vi "4_2_PTLF_Classification_Inference(FPGA).vi"() -> ()   [LabVIEW 2020]
uses:
  <vilib>/userDefined/High Color/nirio_resource_hc.ctl
  <vilib>/FPGAPlugInAG/Dynamic/niLvFpga_Download_Dynamic.vi
  <vilib>/FPGAPlugInAG/Dynamic/niLvFpga_Run_Dynamic.vi
  <vilib>/Ngene/DeepLTK FPGA Addon/Toolkit/NNF_Host/API/NNF_Set_Input/NNF_Set_Input(1D_I8).vi
  <vilib>/rvi/interface/nirviMethod/nirviMethod.xnode
  <vilib>/Ngene/Deep Learning Toolkit/Toolkit/Deep_Learning_Toolkit_by_Ngene.lvlib
  <vilib>/measure/NI_MABase.lvlib
  <vilib>/Ngene/DeepLTK FPGA Addon/Toolkit/DeepLTK_FPGA_Addon.lvlib
  <vilib>/ptbypt/NI_PtbyPt.lvlib
panel:
  in  "Force CPU(All)?":bool
  out "error out 2":errorcluster
  out "Inference Time":dbl=0.08973853333413394 format="%#_3p"
  in  "FPGA Bitfile":path=path "D:/Ngene/GitHub/deepltk_fpga_examples/FPGA Bitfiles/NNF_sbRIO_9609_8Cores_120MHz.lvbitx"
  in  "FPGA target":T1="rio://10.0.0.39/RIO0" caption="RIO Device"
  out "Loop Time":dbl=1506.7505208222221 format="%#_3p"
  in  "Scalers File Path":path=path "D:/Ngene/GitHub/deepltk_fpga_examples/3_PTLF_Classification(PXI,sbRIO)/Models/1_PTLF_Classification_Converted/NNF_ptlf_classifier_net_scalers_24_11_21__13_54_07.cfg"
  in  "Position":dbl(slide)=0.4116719242902208 scale=0.0..1.0
  in  "Fault Generation":T2(tab)=enum."Transient"
  in  "scale":sgl(slide)=0.65833336 scale=0.5..0.7
  in  "Duration(#s)":i32(slide)=388 scale=200.0..600.0
  in  "scale":sgl(slide)=1.4484375 scale=1.35..1.5
  in  "Duration(#s)":i32(slide)=403 scale=200.0..600.0
  in  "Duration(#s)":i32(slide)=366 scale=200.0..600.0
  in  "Tau":dbl(slide)=337.5 scale=200.0..600.0
  in  "Frequency":dbl(slide)=1666.6666666666665 scale=1000.0..2000.0
  in  "Amplitude":dbl(slide)=184.375 scale=150.0..200.0
  in  "Offset":sgl(slide)=105.208336 scale=50.0..150.0
  in  "Duration(#s)":i32(slide)=449 scale=200.0..600.0
  out "Predicted Class":string="Transient"
  out "Class Labels":string[](array[string])=["DC Offset", "Interruption", "Normal", "Sag", "Swell", "Transient"]
  out "Generated WaveForm":waveform(sgl)(graph)={"t0"=timestamp(0 s since 1904-01-01), "dt"=1.0, "Y"=array[2000 elements]}
  in  "Weight File Path":path=path "D:/Ngene/GitHub/deepltk_fpga_examples/3_PTLF_Classification(PXI,sbRIO)/Models/1_PTLF_Classification_Converted/NNF_ptlf_classifier_weights_24_11_21__13_54_07.bin"
  in  "Configuration File Path":path=path "D:/Ngene/GitHub/deepltk_fpga_examples/3_PTLF_Classification(PXI,sbRIO)/Models/1_PTLF_Classification_Converted/NNF_ptlf_classifier_net_cfg_24_11_21__13_54_07.cfg"
  out "Class Probabilities":sgl[](array[slide])=[3.9739523e-05, 7.152872e-06, 1.9828617e-07, 5.2368828e-06, 1.1418055e-05, 0.9999362] scale=0.0..1.0
  in  "Stop":bool
  # "Overview: Demonstrates the usage of DeepLTK FPGA Addon for loading the model pretrained for Power Line Fault Classification and running for inference on FPGA.\nRequirements: \n• DeepLTK - Deep Learning Toolkit for LabVIEW (https://www.ngene.co/deep-learning-toolkit-for-labview)\n• DeepLTK FPGA Addon (https://www.ngene.co/deepltk-accelerator-for-fpga)\nInstructions:\nNote: To run the example on an RT target, copy the converted model to the RT target.\n1. Select FPGA target at FPGA Target control. PXI or remote sbRIO FPGA target can be specified.\n2. Provide path to compiled FPGA bitfile at FPGA Bitfile control. A sample is available in the \"Examples\\FPGA Bitfiles\" folder.\n3. Provide paths to .cfg, .bin and scalers.cfg files generated during model conversion or sample from project (located in \"Models\\1_PTLF_Classification_Converted\" folder)\nat Network Configuration File Path, Weight File Path and Scalers File Path controls.\n4. Run the VI\n5. Choose type of the fault and change the parameters and observe the predicted type of the fault.\n6. Press the Stop button to stop the VI.\nMore Examples: https://github.com/ngenehub/deepltk_fpga_examples"
  # "Power Transmission Line Fault Classification - Inference on FPGA"
  # "Copy resource path from NI MAX if needed"
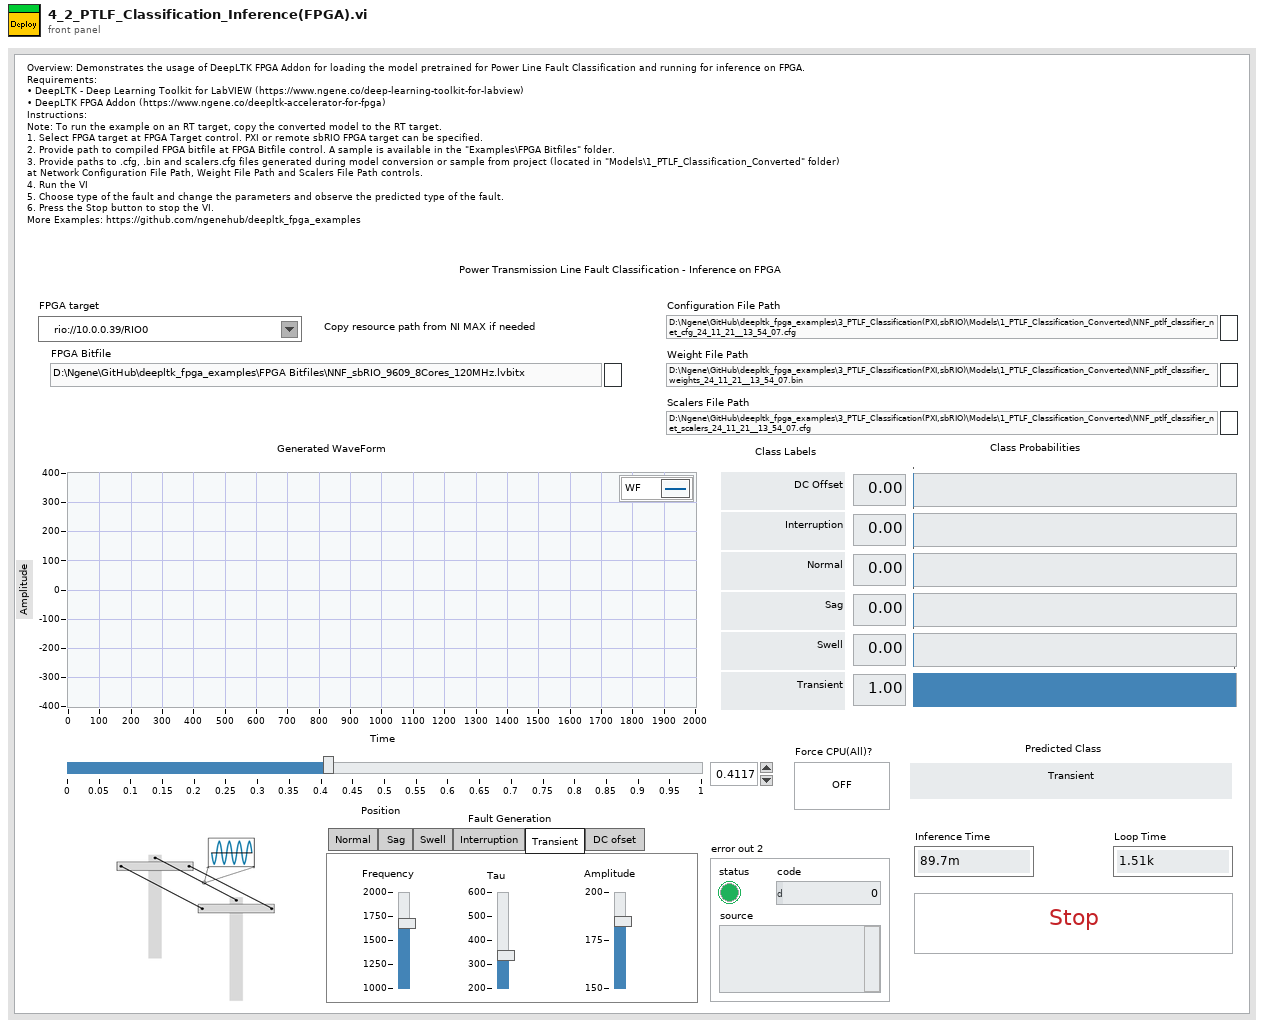
[diagram p1: front panel]
types:
  T1 = typedef "nirio_resource_hc.ctl" = tag
  T2 = enum32{"Normal", "Sag ", "Swell", "Interruption", "Transient", "DC ofset "}
  T3 = typedef "DeepLTK_FPGA_Addon.lvlib/NNF.ctl" = cluster{"FPGA VI Ref ":refnum<k20>, "Subnets":T4[], "Dims_In":T6, "#Cores(enum)":T7, "NN_Ref":T8}
  T4 = typedef "DeepLTK_FPGA_Addon.lvlib/NNF_Subnet.ctl" = cluster{"Subnet Type":T5, "Subnet Data":variant, "Input Scaler":sgl, "Output Scaler":sgl}
  T5 = typedef "DeepLTK_FPGA_Addon.lvlib/NNF_Subnet_Type.ctl" = enum16{"CPU", "FPGA", "Split FPGA"}
  T6 = typedef "Deep_Learning_Toolkit_by_Ngene.lvlib/NN_Dims(C,H,W).ctl" = cluster{"C":i32, "H":i32, "W":i32}
  T7 = typedef "DeepLTK_FPGA_Addon.lvlib/NNF_No_Of_Cores.ctl" = enum16{"4CH", "8CH"}
  T8 = typedef "DeepLTK_FPGA_Addon.lvlib/NN_DVR.ctl" = refnum<data-value>
  T9 = typedef "Deep_Learning_Toolkit_by_Ngene.lvlib/NN_Layer.ctl" = cluster{"Name":string, "Layer_Data":variant, "Layer_Type":T10, "Dims_In":T6, "Layers_In":variant, "Dims_Out":T6, "Layers_Out":variant, "Metrics":T11, "GPU_Data":variant, "mBatch":i32, "NN_Device":T12, "NNg_hdls":T13, "Train?":bool, "Dimty":T14, "RecptField":T15}
  T10 = typedef "Deep_Learning_Toolkit_by_Ngene.lvlib/NN_Layer_Type.ctl" = enum16{"Input1D", "Input3D", "Conv1D", "Conv2D", "Conv2D_Adv", "MaxPool", "AvgPool", "UpSample", "DropOut3D", "ShortCut", "Concat", "SoftMax3D", "FC", "DropOut", "Softmax", "Flatten", "YOLO_v2", "YOLO_v4", "Activation", "BatchNormalization", "Unsupported"}
  T11 = typedef "Deep_Learning_Toolkit_by_Ngene.lvlib/NN_Layer_Metrics.ctl" = cluster{"Data":dbl, "Params":dbl, "Ops":dbl}
  T12 = typedef "Deep_Learning_Toolkit_by_Ngene.lvlib/NN_Device.ctl" = enum16{"CPU", "GPU"}
  T13 = typedef "Deep_Learning_Toolkit_by_Ngene.lvlib/nng_cuda_handles.ctl" = cluster{"cudnn":u64, "cublas":u64, "stream":u64, "curand":u64}
  T14 = typedef "Deep_Learning_Toolkit_by_Ngene.lvlib/NN_Layer_Dimty.ctl" = enum16{"1D", "3D"}
  T15 = typedef "Deep_Learning_Toolkit_by_Ngene.lvlib/NN_Layer_RF_State.ctl" = cluster{"Dims":T16, "J":T16}
  T16 = typedef "Deep_Learning_Toolkit_by_Ngene.lvlib/NN_Dims(V,H).ctl" = cluster{"V":i32, "H":i32}
  T17 = typedef "Deep_Learning_Toolkit_by_Ngene.lvlib/NN.ctl" = cluster{"Name":string, "No of Layers":i32, "mBatch":i32, "Layers":T18[], "Dimty":T19, "Dims_In":T6, "Dims_Out":T6, "Working_Dir":path, "Train?":bool, "Train_Params":T20, "LR_Update_Policy":T23, "Session Data":T25, "Ground_truth":T26, "NNg_hdls":T13, "NN_Device":T12, "GPU Id":i32, "Labels":string[], "Receptive Field":T16[], "Loss_Type":T27, "Loss_Cfg_Prms":variant, "NNG_WS":T28}
  T18 = typedef "Deep_Learning_Toolkit_by_Ngene.lvlib/NN_Layer_ref.ctl" = refnum<data-value>
  T19 = typedef "Deep_Learning_Toolkit_by_Ngene.lvlib/NN_In_Out_Dim-ty.ctl" = enum8{"In1D_Out1D", "In3D_Out1D", "In3D_Out3D", "In3D_OutBBox"}
  T20 = typedef "Deep_Learning_Toolkit_by_Ngene.lvlib/NN_Train_Params.ctl" = cluster{"Optimizer":T21, "Beta_1":sgl, "Beta_2":sgl, "Weight Decay(L1)":sgl, "Weight Decay(L2)":sgl, "Data_Sampling":T22}
  T21 = typedef "Deep_Learning_Toolkit_by_Ngene.lvlib/NN_Train_Optimizer.ctl" = enum16{"SGD", "Adam", "Adagrad", "Adadelta", "RMSProp", "Nesterov"}
  T22 = typedef "Deep_Learning_Toolkit_by_Ngene.lvlib/NN_Train_Data_Sampling.ctl" = enum16{"Random", "Sequential"}
  T23 = typedef "Deep_Learning_Toolkit_by_Ngene.lvlib/NN_LR_Policy_Cfg.ctl" = cluster{"Policy_Type":T24, "LR0":dbl, "k":sgl, "WarmUp_Policy":enum16{"Step", "Ramp"}, "WarmUp_Iter":i32, "WarmUp_Ratio":sgl}
  T24 = typedef "Deep_Learning_Toolkit_by_Ngene.lvlib/NN_LR_Policy_Type.ctl" = enum16{"Manual", "Step", "Exp", "1/t"}
  T25 = typedef "Deep_Learning_Toolkit_by_Ngene.lvlib/NN_Train_Session_Data.ctl" = cluster{"Epochs":sgl, "Tot_Iter":i32, "LR":sgl, "LR_iter":i32}
  T26 = typedef "Deep_Learning_Toolkit_by_Ngene.lvlib/NN_Ground_truth.ctl" = cluster{"Y":variant}
  T27 = typedef "Deep_Learning_Toolkit_by_Ngene.lvlib/NN_Loss_Type.ctl" = enum16{"None", "MSE", "CrossEntropy", "YOLO_v2", "YOLO_v4"}
  T28 = typedef "Deep_Learning_Toolkit_by_Ngene.lvlib/NNG_WS.ctl" = cluster{"NNG_WS_Mem":T29, "Max_WS_Size":i64}
  T29 = typedef "Deep_Learning_Toolkit_by_Ngene.lvlib/NNg_WS_Mem_DVR.ctl" = refnum<data-value>
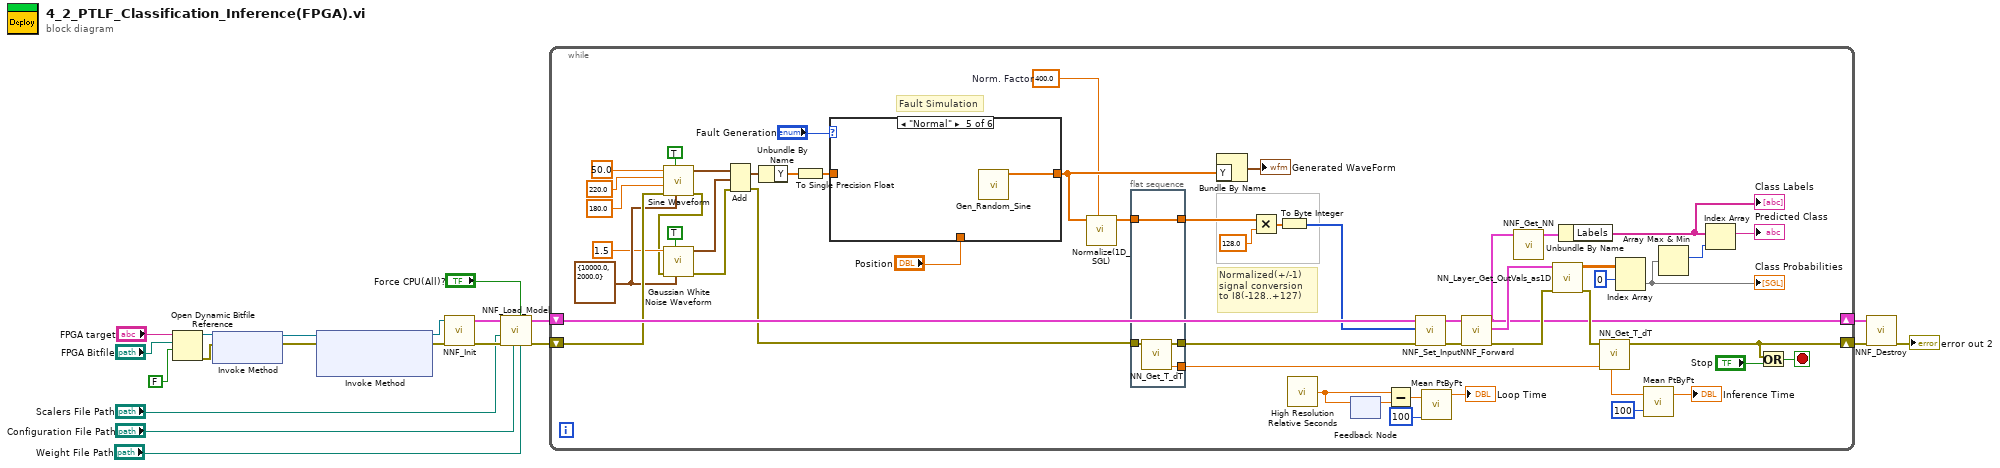
[diagram p0: block diagram]
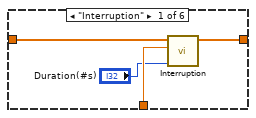
[diagram p2: hidden frame]
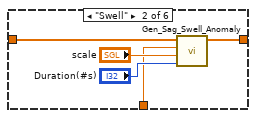
[diagram p3: hidden frame]
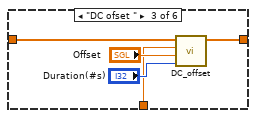
[diagram p4: hidden frame]
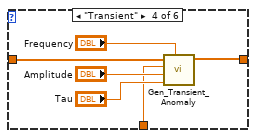
[diagram p5: hidden frame]
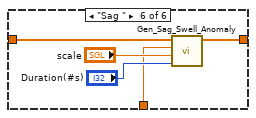
[diagram p6: hidden frame]
diagram:
  n1 = Open Dynamic Bitfile Reference(0:"FPGA target", 1:"FPGA Bitfile", 2:FALSE ("Run When Loaded")) -> (5:w14:refnum<k20>, 8:w9:errorcluster)  [unwired: 2 in]
  n2 = xnode "Invoke Method"("FPGA VI Reference In"=w14, "error in"=w9) -> ("FPGA VI Reference Out"=w13:refnum<k20>, "error out"=w12:errorcluster)
  n3 = xnode "Invoke Method"("FPGA VI Reference In"=w13, "error in"=w12) -> ("FPGA VI Reference Out"=w11:refnum<k20>, "error out"=w10:errorcluster)  [unwired: 1 in]
  n4 = call <vilib>:"NNF_Init.vi"("error in"=w10, "FPGA Interface"=w11) -> ("error out"=w18:errorcluster, "NNF out"=w17:T3)  [unwired: 7 in, 1 out]
  n5 = call <vilib>:"NNF_Load_Model.vi"("Weight File Path"="Weight File Path", "Force CPU(All)?"="Force CPU(All)?", "Network CFG File Path"="Configuration File Path", "Error in"=w18, "Scalers"="Scalers File Path", "NNF in"=w17) -> ("error Out"=w7:errorcluster, "NNF out"=w8:T3)  [unwired: 4 in]
  n6 = while {
    shift-right: [w30] -> w20
    shift-left: w7 -> [w54]
    shift-right: [w23] -> w19
    shift-left: w8 -> [w67]
    stop <- w31 stop-if-true
    w38 = sgl 400.0  # Norm. Factor
    w52 = cluster{"Fs":dbl, "#s":dbl} {"Fs"=10000.0, "#s"=2000.0} ("sampling info")
    # "Normalized(+/-1) signal conversion\nto I8(-128..+127)"
    # "Fault Simulation"
    n7 = call <vilib>:"Sine Waveform.vi"("sampling info"=w52, "reset signal"=TRUE, "error in (no error)"=w54, "phase"=180.0, "amplitude"=220.0, "frequency"=50.0) -> ("error out"=w48:errorcluster, "signal out"=w62:waveform(dbl))  [unwired: 4 in]
    n8 = call <vilib>:"Gaussian White Noise Waveform.vi"("sampling info"=w52, "reset signal"=TRUE, "error in (no error)"=w48, "standard deviation"=sgl 1.5 ("Noise Standart Deviation")) -> ("error out"=w47:errorcluster, "signal out"=w37:waveform(dbl))  [unwired: 6 in]
    n9 = Add(1:w37, 2:w62, 4:w47) -> (0:w50:waveform(dbl), 3:w33:errorcluster)
    n10 = Unbundle By Name(w50) -> ("Y"=w61:dbl[])
    n11 = To Single Precision Float(number=w61) -> (single precision float=w58:sgl[])
    n12 = case shown="\"Normal\"" "Fault Generation" {
      tunnel: [w80 w83 w88 w96 w98 w100] -> w45
      tunnel: w58 -> [w81 w86 w91 w97 _ w103]
      tunnel: "Position" -> [w79 w82 w87 w92 _ w99]
      frame "Interruption" {
        n13 = call "Interruption.vi"("Duration"="Duration(#s)", "Position"=w79, "Sine"=w81) -> ("Sine+Anomaly"=w80:sgl[])  [unwired: 8 in]
      }
      frame "Swell" {
        n14 = call "Gen_Sag_Swell_Anomaly.vi"("Duration"="Duration(#s)", "Amplitude"="scale", "Position"=w82, "Sine"=w86) -> ("Sine+Anomaly"=w83:sgl[])  [unwired: 7 in]
      }
      frame "DC ofset " {
        n15 = call "DC_offset.vi"("Duration"="Duration(#s)", "Ampltude"="Offset", "Position"=w87, "Sine"=w91) -> ("Sine+Anomaly"=w88:sgl[])  [unwired: 7 in]
      }
      frame "Transient" {
        n16 = call "Gen_Transient_Anomaly.vi"("Frequency"="Frequency", "Tau"="Tau", "Amplitude"="Amplitude", "Position"=w92, "Sine"=w97) -> ("Sine+Anomaly"=w96:sgl[])  [unwired: 6 in]
      }
      frame "Normal" {
        n17 = call "Gen_Random_Sine.vi"() -> ("data"=w98:sgl[])  [unwired: 11 in]
      }
      frame "Sag " {
        n18 = call "Gen_Sag_Swell_Anomaly.vi"("Duration"="Duration(#s)", "Amplitude"="scale", "Position"=w99, "Sine"=w103) -> ("Sine+Anomaly"=w100:sgl[])  [unwired: 7 in]
      }
    }
    n19 = call "Normalize(1D_SGL).vi"("Norm. Factor"=w38, "Data In"=w45) -> ("Normalized Out"=w27:sgl[])  [unwired: 9 in]
    n20 = flat-sequence {
      tunnel: [w77] -> w36
      tunnel: [w76] -> w34
      tunnel: w33 -> [w75]
      tunnel: w27 -> [w74]
      tunnel: [w74] -> w26
      frame #0 {
        n21 = call <vilib>:"NN_Get_T_dT.vi"("error in (no error)"=w75) -> ("T_out"=w76:dbl, "error out"=w77:errorcluster)  [unwired: 6 in, 1 out]
      }
    }
    n22 = Bundle By Name("Y"=w45) -> (→"Generated WaveForm":waveform(sgl))  [unwired: 1 in]
    n23 = Multiply(x=w26, y=sgl 128.0) -> (x*y=w40:sgl[])
    n24 = To Byte Integer(number=w40) -> (8bit integer=w28:i8[])
    n25 = call <vilib>:"High Resolution Relative Seconds.vi"() -> ("relative seconds"=w41:dbl)
    n26 = feedback #1() -> (w42:dbl)  [unwired: 1 in]
    n27 = feedback-in #1(w41) -> ()
    n28 = Subtract(x=w41, y=w42) -> (x-y=w44:dbl)
    n29 = call-poly <vilib>:"NNF_Set_Input.vi"("error in"=w36, "Data_in(1D_I8)"=w28, "NNF In"=w67) -> ("error out"=w72:errorcluster, "NNF out"=w71:T3)  [unwired: 7 in]
    n30 = call <vilib>:"Mean PtByPt.vi"("x"=w44, "sample length"=100) -> ("mean"=→"Loop Time":dbl)  [unwired: 2 in, 1 out]
    n31 = call <vilib>:"NNF_Forward.vi"("error in"=w72, "NNF in"=w71) -> ("error out"=w35:errorcluster, "Last_Layer"=w46:T9, "NNF out"=w23:T3)  [unwired: 7 in]
    n32 = call "NNF_Get_NN.vi"("NNF in"=w23) -> ("NN out"=w22:T17)  [unwired: 10 in]
    n33 = call <vilib>:"NN_Layer_Get_OutVals_as1D.vi"("error in (no error)"=w35, "Layer"=w46) -> ("error out"=w73:errorcluster, "Out(as1D)"=w70:sgl[][])  [unwired: 8 in]
    n34 = Unbundle By Name(w22) -> ("Labels"=w21:string[])
    "Class Labels" <- w21
    n35 = call <vilib>:"NN_Get_T_dT.vi"("T_in"=w34, "error in (no error)"=w73) -> ("error out"=w30:errorcluster, "dT"=w32:dbl)  [unwired: 5 in, 1 out]
    n36 = Index Array(array=w70, index (row)=0) -> (element=w66:sgl[])  [unwired: 1 in]
    "Class Probabilities" <- w66
    n37 = call <vilib>:"Mean PtByPt.vi"("x"=w32, "sample length"=100) -> ("mean"=→"Inference Time":dbl)  [unwired: 2 in, 1 out]
    n38 = Array Max & Min(array=w66) -> (max index (indices)=w65:i32)  [unwired: 3 out]
    n39 = Index Array(array=w21, index=w65) -> (element=→"Predicted Class":string)
    n40 = Or(x=w30, y="Stop") -> (x .or. y?=w31:bool)
  }
  n41 = call <vilib>:"NNF_Destroy.vi"("error in"=w20, "NNF in"=w19) -> ("error out"=→"error out 2":errorcluster)  [unwired: 8 in, 1 out]
